vi "Query Macro.vi"(8 "error in (no error)":errorcluster, 10 "Macro Label (\"Label\")":string="Label", 11 "VISA resource name":refnum<visa-resource-name>) -> (0 "error out":errorcluster, 2 "Macro Sequence":string, 3 "VISA resource name out":refnum<visa-resource-name>)   [LabVIEW 2015, in "Rohde&Schwarz CMXP Base.lvlib"]
doc: "Returns the contents of a macro.\n\nAttribute:\n-\n\nRemote-control command:\n*GMC?"
uses:
  <instrlib>/Rohde&Schwarz CMXP Base/Rohde&Schwarz CMXP Base.lvlib
  <instrlib>/Rohde&Schwarz CMXP Base/Private/rsidr_core.llb/rsidr_core.lvlib
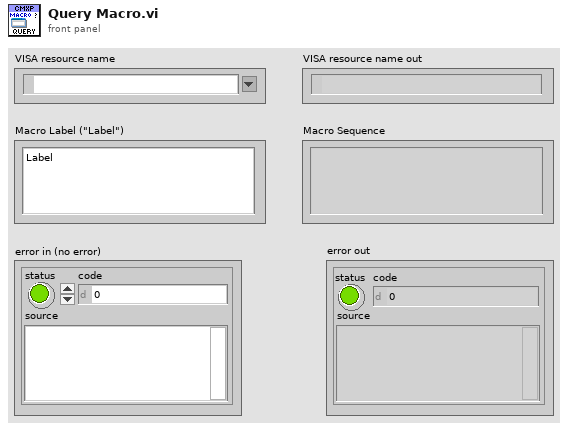
[diagram p1: front panel]
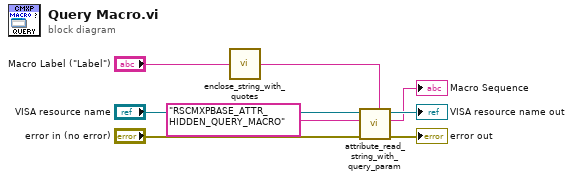
[diagram p0: block diagram]
diagram:
  n1 = call <instrlib>:"enclose_string_with_quotes.vi"("String to enclose"="Macro Label (\"Label\")") -> ("String out"=w1:string)  [unwired: 4 in]
  n2 = call <instrlib>:"attribute_read_string_with_query_param.vi"("Query Parameter (None)"=w1, "error in"="error in (no error)", "Attribute ID"="RSCMXPBASE_ATTR_HIDDEN_QUERY_MACRO", "VISA resource name"="VISA resource name") -> ("error out"=→"error out":errorcluster, "String out"=→"Macro Sequence":string, "VISA resource name out"=→"VISA resource name out":refnum<visa-resource-name>)  [unwired: 5 in]
